vi "Start Sequence.vi"(8 "error in (no error)":errorcluster, 10 "#to save":u16=150 caption="ImgNr.", 11 "POLARIS Target Focus Actor in":refnum<class "POLARIS Target Focus Actor.lvclass">) -> (0 "error out":errorcluster, 3 "POLARIS Target Focus Actor out":refnum<class "POLARIS Target Focus Actor.lvclass">)   [LabVIEW 2014, in "POLARIS Target Focus Actor.lvlib" / "POLARIS Target Focus Actor.lvclass"]
uses:
  POLARIS Target Focus Actor.lvclass
  POLARIS Target Focus Actor.lvclass/POLARIS Target Focus Actor.ctl
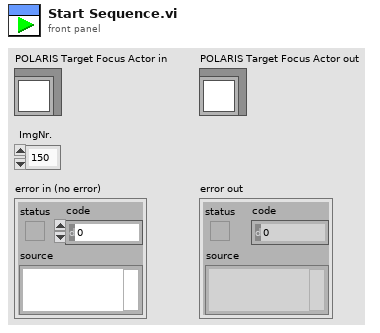
[diagram p1: front panel]
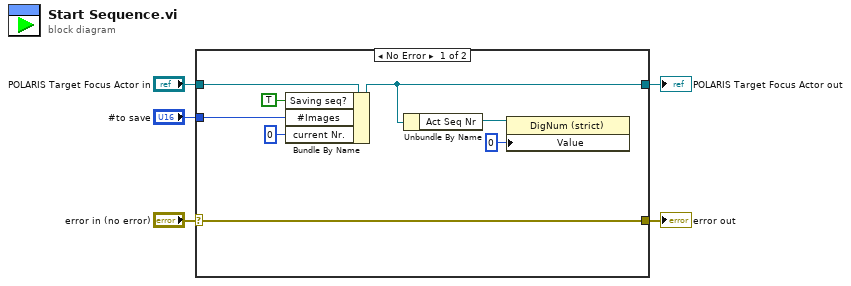
[diagram p0: block diagram]
diagram:
  n1 = case shown="No Error" "error in (no error)" {
    selector: "error in (no error)" -> [w12 w15]
    tunnel: [w12 w15] -> w4
    tunnel: [w9 w14] -> w2
    tunnel: "POLARIS Target Focus Actor in" -> [w13 w14]
    tunnel: "#to save" -> [w10 _]
    frame No Error {
      n2 = Bundle By Name(cluster=w13, "Saving seq?"=TRUE, "#Images"=w10, "current Nr."=u16 0) -> (w9:refnum<class "POLARIS Target Focus Actor.lvclass">)
      n3 = Unbundle By Name(w9) -> ("Act Seq Nr"=w8:refnum<vi>)
      n4 = property class="DigNum (strict)"(reference=w8, "Value"=u16 0) -> ()  [unwired: 1 in, 2 out]
    }
    frame Error {
    }
  }
  "error out" <- w4
  "POLARIS Target Focus Actor out" <- w2
